vi "固定站总磷测量流程.vi"(11 "控制命令":T1(ring)) -> ()   [LabVIEW 2016, in "斯坦道总磷.lvlib"]
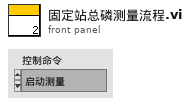
[diagram p1: front panel]
types:
  T1 = enum16{"启动测量", "标样核查", "零点核查", "跨度核查", "空白测试", "平行样测试", "加标回收", "空白校准", "标样校准", "初始化（清洗）", "停止测试", "仪器重启", "校时", "模式设置", "测量间隔设置"}
  T2 = cluster{"仪器":enum16{"", "氨氮", "总磷", "总氮", "CODMn", "CODCr"}, "启动命令":enum16{"启动水样流程", "启动加标流程", "排液", "停止", "柱塞泵启动"}}
  T3 = cluster{"时间标识":timestamp, "设备":string, "日志信息":string, "备注":string}
  T4 = cluster{"时间标识":timestamp, "设备":string, "日志信息":string, "流程参数":string}
  T5 = cluster{"站号":u16, "量程切换":enum32{"H", "L", "AUTO"}, "控制命令":enum16{"启动测量", "标样核查", "零点核查", "跨度核查", "空白测试", "平行样测试", "加标回收", "空白校准", "标样校准", "初始化（清洗）", "停止测试", "仪器重启", "校时", "模式设置", "测量间隔设置"}, "模式设置":enum16{"待机", "连续模式", "周期模式", "定点模式", "受控模式", "手动模式"}, "测量间隔":u16}
  T6 = cluster{"系统时间":timestamp, "工作状态":enum16{"空闲", "水样测试", "标样核查", "零点核查", "跨度核查", "空白测试", "平行样测试", "加标回收", "空白校准", "标样校准", "初始化（清洗）"}, "测量模式":enum16{"待机", "连续模式", "周期模式", "定点模式", "受控模式", "手动模式"}, "告警代码":u16, "故障代码":u16, "日志代码":u16, "软件版本":u16, "F0":sgl, "F1":sgl, "F2":sgl, "F3":sgl, "T":sgl, "H":sgl, "id":u16, "flowid":u16, "量程":u16, "总磷控温温度1":sgl, "营养盐控温温度2":sgl, "ADC":sgl}
  T7 = cluster{"水样测试量程模式":enum16{"H", "L", "AUTO"}, "空白核查量程模式":enum16{"H", "L", "AUTO"}, "跨度核查量程模式":enum16{"H", "L", "AUTO"}, "加标回收量程模式":enum16{"H", "L", "AUTO"}}
  T8 = enum16{"空闲", "水样测试", "标样核查", "零点核查", "跨度核查", "空白测试", "平行样测试", "加标回收", "空白校准", "标样校准", "初始化（清洗）"}
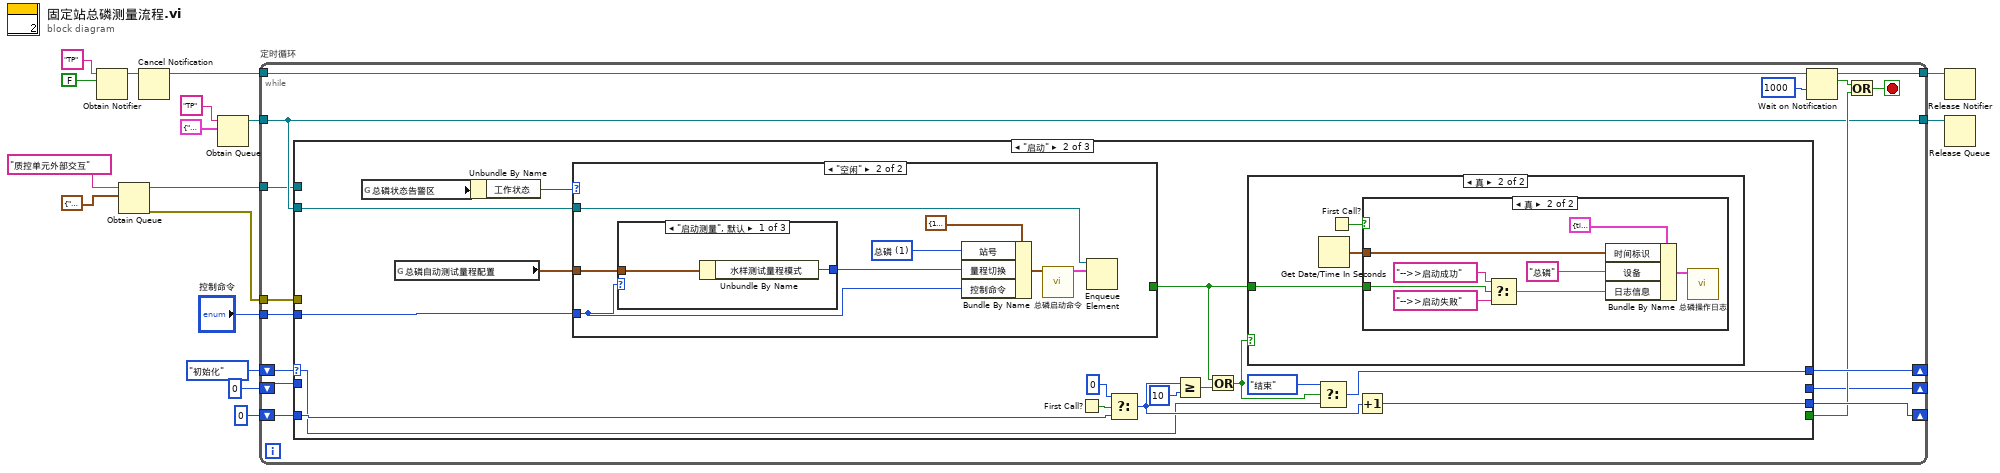
[diagram p0: block diagram]
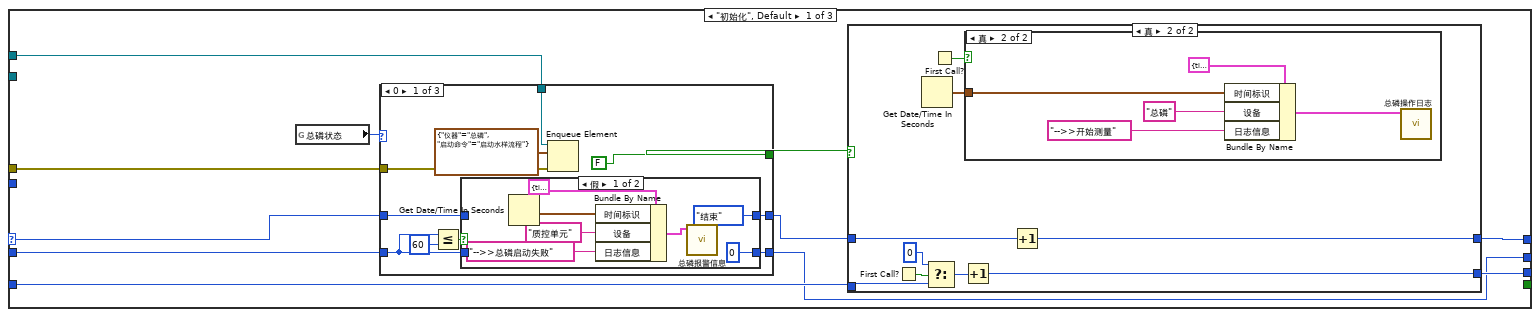
[diagram p2: hidden frame]
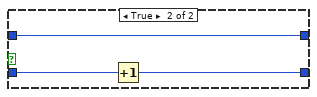
[diagram p3: hidden frame]
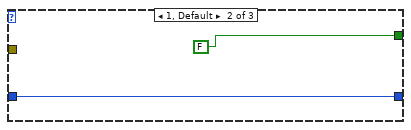
[diagram p4: hidden frame]
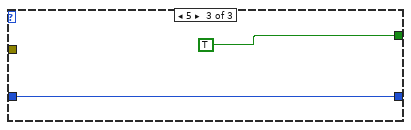
[diagram p5: hidden frame]
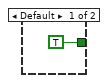
[diagram p10: hidden frame]
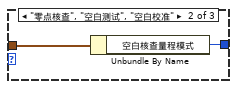
[diagram p11: hidden frame]
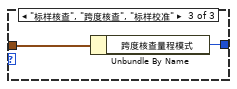
[diagram p12: hidden frame]
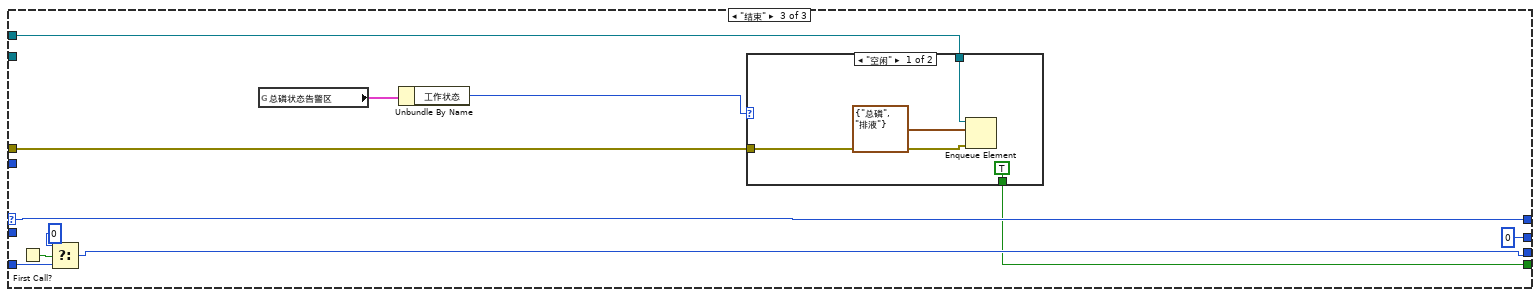
[diagram p13: hidden frame]
diagram:
  n1 = Obtain Notifier(name (unnamed)="TP" ("名称（未命名）"), notification data type=FALSE) -> (notifier out=w12:refnum<notifier>)  [unwired: 2 in, 2 out]
  n2 = Obtain Queue(name (unnamed)="质控单元外部交互" ("名称（未命名）"), element data type=T2 {"仪器"=enum."氨氮", "启动命令"=enum."启动水样流程"} ("元素")) -> (queue out=w3:refnum<queue>, error out=w2:errorcluster)  [unwired: 3 in, 1 out]
  n3 = Cancel Notification(0:w12) -> (8:w11:refnum<notifier>)  [unwired: 1 in, 2 out]
  n4 = Obtain Queue(name (unnamed)="TP" ("名称（未命名）"), element data type=cluster{"命令":string, "data":variant} {"命令"="", "data"=variant}) -> (queue out=w15:refnum<queue>)  [unwired: 3 in, 2 out]
  n5 = while "定时循环" {
    tunnel: w15 -> [w22]
    tunnel: w11 -> [w33]
    tunnel: "控制命令" -> [w28]
    shift-right: [w27] -> _
    shift-left: enum16{"初始化", "启动", "结束"}."初始化" -> [w29]
    shift-right: [w25] -> _
    shift-left: 0 -> [w26]
    tunnel: [w23] -> w7
    tunnel: [w22] -> w8
    tunnel: w3 -> [w21]
    tunnel: w2 -> [w20]
    shift-right: [w18] -> _
    shift-left: 0 -> [w19]
    stop <- w30 stop-if-true
    n6 = case shown="\"启动\"" w29 {
      selector: w29 -> [w37 w90 w138]
      tunnel: w28 -> [_ w101 _]
      tunnel: w22 -> [_ w100 _]
      tunnel: [w44 w91 w138] -> w27
      tunnel: w26 -> [w43 w95 w135]
      tunnel: [w42 w94 w134] -> w25
      tunnel: [_ _ w129] -> w24
      tunnel: w21 -> [w39 _ w133]
      tunnel: w20 -> [w38 _ w132]
      tunnel: w19 -> [w35 _ _]
      tunnel: [w34 _ 0] -> w18
      frame "初始化", Default {
        n7 = global read "VAR总磷全局变量.vi" "总磷状态"() -> (w40:u16)
        n8 = case shown="0" w40 {
          tunnel: [FALSE ("s") FALSE ("s") TRUE ("s")] -> w41
          tunnel: w39 -> [w53 _ _]
          tunnel: w38 -> [w52 _ _]
          tunnel: w37 -> [w48 w65 w67]
          tunnel: [w47 w65 w67] -> w36
          tunnel: w35 -> [w46 _ _]
          tunnel: [w45 _ _] -> w34
          frame 0 {
            n9 = Less Or Equal?(x=w46, y=60) -> (x <= y?=w49:bool)
            n10 = case shown="假" w49 {
              tunnel: w46 -> [_ w64]
              tunnel: [0 w63] -> w45
              tunnel: w48 -> [_ w62]
              tunnel: [enum16{"初始化", "启动", "结束"}."结束" w62] -> w47
              frame False {
                n11 = Get Date/Time In Seconds() -> (seconds since 1Jan1904=w57:timestamp)
                n12 = Bundle By Name(cluster=T3 {"时间标识"=timestamp(0 s since 1904-01-01), "设备"="", "日志信息"="", "备注"=""} ("data in"), "时间标识"=w57, "设备"="质控单元", "日志信息"="-->>总磷启动失败") -> (w56:T3)
                n13 = call "总磷报警信息.vi"("data in"=w56) -> ()  [unwired: 10 in, 1 out]
              }
              frame True {
                n14 = Increment(x=w64) -> (x+1=w63:i32)
              }
            }
            n15 = Enqueue Element(queue=w53, element=T2 {"仪器"=enum."总磷", "启动命令"=enum."启动水样流程"} ("元素"), error in (no error)=w52) -> ()  [unwired: 1 in, 3 out]
          }
          frame 1, Default {
          }
          frame 5 {
          }
        }
        n16 = case shown="真" w41 {
          tunnel: w36 -> [w70 w77]
          tunnel: [w70 w76] -> w44
          tunnel: w43 -> [w69 w74]
          tunnel: [w69 w71] -> w42
          frame False {
          }
          frame True {
            n17 = First Call?() -> (First Call?: T/F=w75:bool)
            n18 = Get Date/Time In Seconds() -> (seconds since 1Jan1904=w79:timestamp)
            n19 = Select(t=0, s=w75, f=w74) -> (s? t:f=w72:i32)
            n20 = First Call?() -> (First Call?: T/F=w78:bool)
            n21 = Increment(x=w72) -> (x+1=w71:i32)
            n22 = case shown="真" w78 {
              tunnel: w79 -> [_ w83]
              frame False {
              }
              frame True {
                n23 = Bundle By Name(cluster=T4 {"时间标识"=timestamp(0 s since 1904-01-01), "设备"="", "日志信息"="", "流程参数"=""} ("data in"), "时间标识"=w83, "设备"="总磷", "日志信息"="-->>开始测量") -> (w84:T4)
                n24 = call "总磷操作日志.vi"("data in"=w84) -> ()  [unwired: 11 in]
              }
            }
            n25 = Increment(x=w77) -> (x+1=w76:enum16{"初始化", "启动", "结束"})
          }
        }
      }
      frame "启动" {
        n26 = global read "VAR总磷全局变量.vi" "总磷状态告警区"() -> (w99:T6)
        n27 = global read "总磷断电保存全局变量.vi" "总磷自动测试量程配置"() -> (w85:T7)
        n28 = Unbundle By Name(w99) -> ("工作状态"=w98:T8)
        n29 = case shown="\"空闲\"" w98 {
          tunnel: w85 -> [_ w119]
          tunnel: w101 -> [_ w114]
          tunnel: w100 -> [_ w118]
          tunnel: [TRUE _] -> w86
          frame Default {
          }
          frame "空闲" {
            w117 = u16 1 items=["总磷"=1, "总氮"=2, "氨氮"=3] ("站号")
            n30 = case shown="\"启动测量\", 默认" w114 {
              tunnel: w119 -> [w123 w125 w127]
              tunnel: [w122 w124 w126] -> w121
              frame "启动测量", Default {
                n31 = Unbundle By Name(w123) -> ("水样测试量程模式"=w122:enum16{"H", "L", "AUTO"})
              }
              frame "零点核查", "空白测试", "空白校准" {
                n32 = Unbundle By Name(w125) -> ("空白核查量程模式"=w124:enum16{"H", "L", "AUTO"})
              }
              frame "标样核查", "跨度核查", "标样校准" {
                n33 = Unbundle By Name(w127) -> ("跨度核查量程模式"=w126:enum16{"H", "L", "AUTO"})
              }
            }
            n34 = Bundle By Name(cluster=T5 {"站号"=1, "量程切换"=enum."AUTO", "控制命令"=enum."启动测量", "模式设置"=enum."待机", "测量间隔"=0} ("参数"), "站号"=w117, "量程切换"=w121, "控制命令"=w114) -> (w115:T5)
            n35 = call "总磷启动命令.vi"("参数"=w115) -> ("启动命令"=w120:cluster{"命令":string, "data":variant})  [unwired: 10 in]
            n36 = Enqueue Element(queue=w118, element=w120) -> ()  [unwired: 2 in, 3 out]
          }
        }
        n37 = First Call?() -> (First Call?: T/F=w97:bool)
        n38 = Select(t=0, s=w97, f=w95) -> (s? t:f=w93:i32)
        n39 = Greater Or Equal?(x=w93, y=10) -> (x >= y?=w89:bool)
        n40 = Or(x=w86, y=w89) -> (x .or. y?=w87:bool)
        n41 = case shown="真" w87 {
          tunnel: w86 -> [_ w102]
          frame False {
          }
          frame True {
            n42 = Get Date/Time In Seconds() -> (seconds since 1Jan1904=w103:timestamp)
            n43 = First Call?() -> (First Call?: T/F=w104:bool)
            n44 = case shown="真" w104 {
              tunnel: w103 -> [_ w111]
              tunnel: w102 -> [_ w108]
              frame False {
              }
              frame True {
                n45 = Select(t="-->>启动成功" ("日志信息"), s=w108, f="-->>启动失败" ("日志信息")) -> (s? t:f=w105:string)
                n46 = Bundle By Name(cluster=T4 {"时间标识"=timestamp(0 s since 1904-01-01), "设备"="", "日志信息"="", "流程参数"=""} ("data in"), "时间标识"=w111, "设备"="总磷", "日志信息"=w105) -> (w112:T4)
                n47 = call "总磷操作日志.vi"("data in"=w112) -> ()  [unwired: 11 in]
              }
            }
          }
        }
        n48 = Select(t=enum16{"初始化", "启动", "结束"}."结束", s=w87, f=w90) -> (s? t:f=w91:enum16{"初始化", "启动", "结束"})
        n49 = Increment(x=w93) -> (x+1=w94:i32)
      }
      frame "结束" {
        n50 = First Call?() -> (First Call?: T/F=w137:bool)
        n51 = Select(t=0, s=w137, f=w135) -> (s? t:f=w134:i32)
        n52 = global read "VAR总磷全局变量.vi" "总磷状态告警区"() -> (w131:T6)
        n53 = Unbundle By Name(w131) -> ("工作状态"=w130:T8)
        n54 = case shown="\"空闲\"" w130 {
          tunnel: w133 -> [w141 _]
          tunnel: w132 -> [w140 _]
          tunnel: [TRUE _] -> w129
          frame "空闲" {
            n55 = Enqueue Element(queue=w141, element=T2 {"仪器"=enum."总磷", "启动命令"=enum."排液"} ("元素"), error in (no error)=w140) -> ()  [unwired: 1 in, 3 out]
          }
          frame "水样测试", Default {
          }
        }
      }
    }
    n56 = Wait on Notification(notifier=w33, timeout in ms (-1)=1000 ("超时毫秒(-1)")) -> (notifier out=w23:refnum<notifier>, notification=w31:bool)  [unwired: 2 in, 2 out]
    n57 = Or(x=w31, y=w24) -> (x .or. y?=w30:bool)
  }
  n58 = Release Notifier(notifier=w7) -> ()  [unwired: 2 in, 3 out]
  n59 = Release Queue(queue=w8) -> ()  [unwired: 2 in, 3 out]
